vi "UHR-Fleezers Control (host) - 16.2.2v2.vi"() -> ()   [LabVIEW 2014] (continued)
            n3715 = Concatenate Strings("Lost tether (" ("Message to add"), w5032, " s)." ("string")) -> (w5034:string)
            n3716 = local write "Tether"(FALSE ("Tether")) -> ()
            n3717 = call "Update messages.vi"("Message to add"=w5034, "Old message string"=w5039) -> ("New message string"=w5038:string)
            n3718 = local write "Messages"(w5038) -> ()
            n3719 = property on="Fl. Triggered..." class="Bool (strict)"("Val(Sgnl)"=w5030) -> ()  [unwired: 2 in, 2 out]
            n3720 = local write "Dip for Protein"(w5030) -> ()
            n3721 = property on="Trap Pos. FB ON" class="Bool (strict)"("Val(Sgnl)"=w5030) -> ()  [unwired: 2 in, 2 out]
            n3722 = property on="Trap Trig. Fl." class="Bool (strict)"("Val(Sgnl)"=w5030) -> ()  [unwired: 2 in, 2 out]
          }
        }
      }
    }
    n3723 = case "For triggering actions based on the trap position (e.g., turning the excitation laser on if trap under feedback moves so far)" shown="True" "Trap Trig. Fl." {
      tunnel: w4490 -> [_ w4918]
      tunnel: w4503 -> [_ w4917]
      tunnel: ["" ("t") w4916] -> w4511
      tunnel: w4495 -> [_ w4915]
      tunnel: [0 ("t") w4914] -> w4508
      tunnel: w4507 -> [_ w4913]
      tunnel: w4482 -> [_ w4912]
      tunnel: w4481 -> [_ w4911]
      frame False {
      }
      frame True {
        n3724 = case shown="\"Wait for trigger\"" w4917 {
          tunnel: w4918 -> [w4935 _ _ w4983]
          tunnel: [w4932 w4964 "" ("t") w4986] -> w4916
          tunnel: w4915 -> [_ _ _ w4974]
          tunnel: [w4931 w4961 0 ("t") w4975] -> w4914
          tunnel: w4913 -> [_ w4963 _ w4981]
          tunnel: w4912 -> [w4920 w4958 _ w4977]
          tunnel: w4911 -> [w4919 w4957 _ w4976]
          frame "Wait for trigger" {
            n3725 = local read "Trap Trig. (FPGA)"() -> (w4923:bool)
            n3726 = Subtract(x=w4935, y="Mean T1 Position\nto compare (nm)") -> (x-y=w4928:dbl[])
            n3727 = call <vilib>:"Std Deviation and Variance.vi"("X"=w4928) -> ("mean"=→"mean":dbl, "standard deviation"=→"standard\ndeviation":dbl)  [unwired: 1 in, 1 out]
            n3728 = Array Max & Min(array=w4928) -> (max value=→"max value":dbl, min value=→"min value":dbl)  [unwired: 2 out]
            n3729 = Greater?(x=w4928, y="Threshold (nm)") -> (0:w4938:bool[])
            n3730 = case shown="True" w4923 {
              tunnel: w4920 -> [_ w4944]
              tunnel: w4919 -> [_ w4943]
              tunnel: [FALSE ("TTrig?") w4942] -> w4926
              frame False {
              }
              frame True {
                n3731 = xnode "Read/Write Control"("FPGA VI Reference In"=w4944, "error in"=w4943) -> ("TTrig?"=w4942:bool)  [unwired: 2 out]
              }
            }
            n3732 = Or Array Elements(Boolean array=w4938) -> (logical OR=w4925:bool)
            n3733 = Select(t=w4926, s=w4923, f=w4925) -> (s? t:f=w4924:bool)
            n3734 = Not(x=w4923) -> (.not. x?=w4922:bool)
            n3735 = And(x=w4924, y=w4922) -> (x .and. y?=w4921:bool)
            n3736 = Select(t="Triggered", s=w4924, f="Wait for trigger") -> (s? t:f=w4932:string)
            n3737 = case shown="True" w4924 {
              tunnel: [0 0] -> w4931
              tunnel: w4920 -> [_ w4949]
              tunnel: w4919 -> [_ w4948]
              frame False {
                "Waiting" <- TRUE ("Waiting")
              }
              frame True {
                n3738 = xnode "Read/Write Control"("FPGA VI Reference In"=w4949, "error in"=w4948, "TTrig?"=FALSE) -> ()  [unwired: 2 out]
                n3739 = local read "Messages"() -> (w4952:string)
                n3740 = call <vilib>:"Beep.vi"() -> ()  [unwired: 12 in]
                n3741 = call "Update messages.vi"("Message to add"="Unwinding trigger.", "Old message string"=w4952) -> ("New message string"=w4953:string)
                n3742 = local write "Messages"(w4953) -> ()
                n3743 = local write "Waiting"(FALSE ("Waiting")) -> ()
                "Triggered" <- TRUE ("Triggered")
              }
            }
            n3744 = case "Only need to turn on laser if host triggered" shown="True" w4921 {
              frame False {
              }
              frame True {
                n3745 = property on="Green Laser ON" class="Bool (strict)"("Val(Sgnl)"=TRUE ("Value (Signaling)")) -> ()  [unwired: 2 in, 2 out]
              }
            }
          }
          frame "Triggered" {
            n3746 = local read "Trap Trig. (FPGA)"() -> (w4960:bool)
            n3747 = Increment(x=w4963) -> (x+1=w4961:i32)
            n3748 = Greater Or Equal?(x=w4961, y="Fl. ON time (n)") -> (x >= y?=w4959:bool)
            n3749 = Select(t="Wait for trigger", s=w4959, f="Triggered" ("t")) -> (s? t:f=w4964:string)
            n3750 = And(x=w4959, y=w4960) -> (x .and. y?=w4956:bool)
            n3751 = case shown="True" w4956 {
              tunnel: w4958 -> [_ w4968]
              tunnel: w4957 -> [_ w4967]
              frame False {
              }
              frame True {
                n3752 = xnode "Read/Write Control"("FPGA VI Reference In"=w4968, "error in"=w4967, "FPGA Trap Trig"=TRUE) -> ()  [unwired: 2 out]
              }
            }
            n3753 = case shown="True" w4959 {
              frame False {
              }
              frame True {
                w4970 = FALSE ("Value (Signaling)")
                n3754 = local write "Triggered"(w4970) -> ()
                n3755 = local write "Waiting"(TRUE ("Waiting")) -> ()
                n3756 = property on="Green Laser ON" class="Bool (strict)"("Val(Sgnl)"=w4970) -> ()  [unwired: 2 in, 2 out]
              }
            }
          }
          frame "Do nothing" {
          }
          frame "Initialize", Default {
            n3757 = Increment(x=w4981) -> (x+1=w4985:i32)
            n3758 = Select(t=1, s=w4974, f=w4985) -> (s? t:f=w4975:i32)
            n3759 = feedback #29(w4983) -> (w4989:dbl[])
            n3760 = Build Array (concatenate)(w4983, w4989) -> (w4982:dbl[])
            n3761 = Greater Or Equal?(x=w4975, y="Wait to get offset (n)") -> (x >= y?=w4978:bool)
            n3762 = Select(t=w4983, s=w4974, f=w4982) -> (s? t:f=w4984:dbl[])
            n3763 = feedback-in #29(w4984) -> ()
            n3764 = call-poly <vilib>:"Mean.vi"("X"=w4984) -> ("mean"=w4979:dbl)  [unwired: 1 out]
            n3765 = local write "Mean T1 Position\nto compare (nm)"(w4979) -> ()
            n3766 = case shown="True" w4974 {
              tunnel: w4977 -> [_ w4995]
              tunnel: w4976 -> [_ w4994]
              frame False {
              }
              frame True {
                w4991 = FALSE ("FPGA Trap Trig")
                n3767 = xnode "Read/Write Control"("FPGA VI Reference In"=w4995, "error in"=w4994, "FPGA Trap Trig"=w4991) -> ("FPGA VI Reference Out"=w4993:T25, "error out"=w4992:errorcluster)
                n3768 = xnode "Read/Write Control"("FPGA VI Reference In"=w4993, "error in"=w4992, "TTrig?"=w4991) -> ()  [unwired: 2 out]
              }
            }
            n3769 = Select(t="Wait for trigger", s=w4978, f="Initialize") -> (s? t:f=w4986:string)
            n3770 = case shown="True" w4978 {
              tunnel: w4979 -> [_ w4998]
              tunnel: w4977 -> [_ w5007]
              tunnel: w4976 -> [_ w5006]
              frame False {
                n3771 = local write "Waiting"(FALSE ("Waiting")) -> ()
                "Initializing" <- TRUE ("Initializing")
              }
              frame True {
                n3772 = local read "Threshold (nm)"() -> (w5010:dbl)
                n3773 = local read "AOM X Cal (nm/MHz)"() -> (w5009:dbl)
                n3774 = Add(x=w4998, y=w5010) -> (x+y=w5011:dbl)
                n3775 = Divide(x=w5011, y=w5009) -> (x/y=w5008:dbl)
                n3776 = call "IR AOM freq to word.vi"("Frequency In (MHz)"=w5008) -> ("Frequency Word Out (double)"=w5005:dbl)
                n3777 = local write "Initializing"(FALSE ("Initializing")) -> ()
                n3778 = local write "Waiting"(TRUE ("Waiting")) -> ()
                n3779 = To Quad Integer(1:w5005) -> (0:w5004:i64)
                n3780 = xnode "Read/Write Control"("FPGA VI Reference In"=w5007, "error in"=w5006, "FPGA TTrig Thresh"=w5004) -> ("FPGA VI Reference Out"=w5001:T25, "error out"=w5000:errorcluster)
                n3781 = xnode "Read/Write Control"("FPGA VI Reference In"=w5001, "error in"=w5000, "FPGA Trap Trig"=TRUE) -> ()  [unwired: 2 out]
              }
            }
          }
        }
      }
    }
    n3782 = feedback-in #27(w4511) -> ()
    n3783 = feedback-in #28(w4508) -> ()
    n3784 = xnode ("Read/Write Control")("FPGA VI Reference In"=w4646, "error in"=w4645) -> ("FPGA VI Reference Out"=w4493:T25, "error out"=w4492:errorcluster, "AI2 Y Sum Set 1"=w4717:i16, "AI2 Y Sum Set 2"=w4716:i16, "AI1 X Set 1"=w4557:fxp<+/-,16,1>, "AI1 X Set 2"=w4556:fxp<+/-,16,1>, "Trap Pos FB Int Signal"=→"Trap Pos FB Int Signal":fxp<+/-,24,9>, "Trap Pos FB Int-Norm Signal"=→"Trap Pos FB Int-Norm Signal":fxp<+/-,16,1>, "Trap Pos FB Action"=w4550:i64, "Scanning"=→"AOD Scanning":bool, "Scan I"=→"AOD Scan I":u64, "Scanning MCL"=w4719:bool, "Scan I (MCL)"=→"MCL Scan I":u64, "Green FB Sum"=w4662:i16, "Trap Pos FB Action"=w4480:i64, "TTrig Fin Thresh"=w4476:i64, "Red FB Intensity"=w4460:i16, "Blue Intensity"=w4455:i16, "Random phase generated"=→"RF phase":fxp<+,14,14>)
    "MCL Scanning" <- w4719
    "Trap Pos FB Action" <- w4550
    n3785 = Divide(x=w4460, y=3276.7) -> (x/y=w4459:dbl)
    "Red laser intensity (V)" <- w4459
    n3786 = Divide(x=w4455, y=3276.7) -> (x/y=w4454:dbl)
    "Blue laser intensity (V)" <- w4454
    n3787 = Divide(x=w4662, y=3276.7) -> (x/y=w4458:dbl)
    "Green laser intensity (V)" <- w4458
    n3788 = local read "FB Trig Integrate"() -> (w4474:u32)
    n3789 = Divide(x=w4480, y=w4474) -> (x/y=w4473:dbl)
    "TTrig Sig (Int)" <- w4473
    n3790 = Bundle(w4458, w4459, w4454) -> (→"Fluorescence laser intensities plot":cluster{dbl, dbl, dbl})  [unwired: 1 in]
    n3791 = Divide(x=w4476, y=w4474) -> (x/y=w4471:dbl)
    "TTrig Fin Thresh (Int)" <- w4471
    n3792 = local read "AOM X Cal (nm/MHz)"() -> (w4479:dbl)
    n3793 = local read "AI2 (V)"() -> (w4718:cluster{"Set 1":dbl, "Set 2":dbl})
    n3794 = Bundle By Name(cluster=w4718, "Set 1"=w4717, "Set 2"=w4716) -> (w4714:cluster{"Set 1":dbl, "Set 2":dbl})
    n3795 = Divide(x=w4550, y=327.67) -> (x/y=→"Action (%)":dbl)
    n3796 = local read "Trap X (AI1)"() -> (w4570:T12)
    n3797 = call "IR AOM word double to freq.vi"("Frequency Word In (double)"=w4471) -> ("Frequency Out (MHz)"=w4470:dbl)
    n3798 = call "IR AOM word double to freq.vi"("Frequency Word In (double)"=w4473) -> ("Frequency Out (MHz)"=w4472:dbl)
    n3799 = Divide(x=w4714, y=3276.7) -> (x/y=w4713:cluster{"Set 1":dbl, "Set 2":dbl})
    n3800 = Multiply(x=w4472, y=w4479) -> (x*y=w4478:dbl)
    "TTrig Sig (nm)" <- w4478
    n3801 = Multiply(x=w4470, y=w4479) -> (x*y=w4477:dbl)
    "TTrig Fin Thresh (nm)" <- w4477
    n3802 = local write "AI2 (V)"(w4713) -> ()
    n3803 = Bundle(cluster=w4570, "Trap 1"=w4557, "Trap 2"=w4556) -> (→"Trap X (AI1)":T12)
    n3804 = Bundle(w4478, w4477) -> (→"TTrig":cluster{dbl, dbl})  [unwired: 1 in]
    n3805 = flat-sequence "To save data" {
      tunnel: [w5878] -> w4737
      tunnel: [w5879] -> w4736
      tunnel: w4690 -> [w5872]
      tunnel: w4498 -> [w5876]
      tunnel: ["Save Calibration"] -> w4710
      tunnel: w4707 -> [w5875]
      tunnel: [w5868] -> w4706
      tunnel: [w5865] -> w4705
      tunnel: [w5862] -> w4704
      tunnel: w4689 -> [w5864]
      tunnel: w4630 -> [w5858]
      tunnel: [w5858] -> w4629
      tunnel: [w5850] -> w4604
      tunnel: [w5853] -> w4538
      tunnel: [w5852] -> w4537
      tunnel: [w5846] -> w4392
      tunnel: w4737 -> [w6158]
      tunnel: w4736 -> [w6157]
      tunnel: w4539 -> [w6156]
      tunnel: w4710 -> [w6155]
      tunnel: w4706 -> [w6153]
      tunnel: w4705 -> [w6152]
      tunnel: w4704 -> [w6151]
      tunnel: w4611 -> [w6150]
      tunnel: w4638 -> [w6149]
      tunnel: w4629 -> [w6148]
      tunnel: w4604 -> [w6147]
      tunnel: w4399 -> [w6146]
      tunnel: w4441 -> [w6145]
      tunnel: w4538 -> [w6144]
      tunnel: w4537 -> [w6143]
      tunnel: w4536 -> [w6142]
      tunnel: w4462 -> [w6141]
      tunnel: w4390 -> [w6140]
      tunnel: w4392 -> [w6139]
      frame #0 {
        n3806 = Or(x="Start Saving", y="Start saving data + video") -> (x .or. y?=w5850:bool)
        n3807 = case shown="True" "Start saving data + video" {
          frame False {
          }
          frame True {
            n3808 = stacked-sequence {
              frame #0 {
                n3809 = local write "New Video File"(TRUE ("New Video File")) -> ()
              }
              frame #1 {
                n3810 = local write "Save Video"(TRUE ("Save Video")) -> ()
              }
            }
          }
        }
        n3811 = Or(x="Save N Sets", y=w5850) -> (x .or. y?=w5859:bool)
        n3812 = To Double Precision Float(number=w5875) -> (double precision float=w5869:dbl)
        n3813 = Build Array(w5859, "Save Calibration", w5872, w5864) -> (w5874:bool[])
        n3814 = Compound Arithmetic op=OR("Save Calibration", w5872, w5859, w5864) -> (w5877:bool)
        n3815 = Boolean Array To Number(Boolean array=w5874) -> (number=w5871:u32)
        n3816 = feedback #30(FALSE ("Save APD Data\nwith Trap Data")) -> (w5854:bool)
        n3817 = feedback #31(refnum<k0> refnum) -> (w5880:refnum<file>)
        n3818 = feedback #32(FALSE ("Save APD Data\nwith Trap Data")) -> (w5863:bool)
        n3819 = feedback #33(0) -> (w5882:i32)
        n3820 = feedback #34() -> (w5870:u32)  [unwired: 1 out]
        n3821 = feedback #35(refnum<k0> refnum) -> (w5847:refnum<file>)
        n3822 = feedback #36(refnum<k0> refnum) -> (w5856:refnum<file>)
        n3823 = feedback #37(refnum<k0> refnum) -> (w5866:refnum<file>)
        n3824 = case shown="True" w5877 {
          tunnel: [w5892 1] -> w5878
          tunnel: w5882 -> [w5894 _]
          tunnel: [w5893 w5927] -> w5879
          tunnel: w5880 -> [w5893 _]
          tunnel: w5876 -> [_ w5945]
          tunnel: w5869 -> [_ w5943]
          tunnel: w5871 -> [_ w5946]
          tunnel: [w5891 w5926] -> w5868
          tunnel: w5870 -> [w5891 _]
          tunnel: [w5890 w5924] -> w5865
          tunnel: w5866 -> [w5890 _]
          tunnel: [w5889 w5923] -> w5862
          tunnel: w5863 -> [w5889 _]
          tunnel: w5850 -> [_ w5921]
          tunnel: w5858 -> [_ w5920]
          tunnel: [w5888 w5912] -> w5852
          tunnel: w5856 -> [w5888 _]
          tunnel: [w5887 w5911] -> w5853
          tunnel: w5854 -> [w5887 _]
          tunnel: [w5886 w5895] -> w5846
          tunnel: w5847 -> [w5886 _]
          frame False {
            n3825 = Increment(x=w5894) -> (x+1=w5892:i32)
          }
          frame True {
            w5917 = FALSE ("Start Saving")
            w5922 = 9.0  # File Version
            w5929 = FALSE ("prepend array or string size? (T)")
            w5928 = T34."big-endian, network order" ("byte order (0:big-endian, network order)")
            # "Save trap position\ndata"
            n3826 = local read "BD 1 Frequency 1 (MHz)"() -> (w5942:dbl)
            n3827 = local read "BD 2 Frequency 1 (MHz)"() -> (w5941:dbl)
            n3828 = local read "BD 1 Frequency 2 (MHz)"() -> (w5940:dbl)
            n3829 = local read "BD 2 Frequency 2 (MHz)"() -> (w5939:dbl)
            n3830 = local read "BD 1 Frequency 3 (MHz)"() -> (w5938:dbl)
            n3831 = local read "BD 2 Frequency 3 (MHz)"() -> (w5937:dbl)
            n3832 = Array Size(array=w5920) -> (size(s)=w5919:i32)
            n3833 = To Double Precision Float(number=w5919) -> (double precision float=w5918:dbl)
            n3834 = local write "Save Calibration"(w5917) -> ()
            n3835 = local write "Start Saving"(w5917) -> ()
            n3836 = Build Array("Save APD Data\nwith Trap Data", "Save Trap Pos. Data") -> (w5914:bool[])
            n3837 = Boolean Array To Number(Boolean array=w5914) -> (number=w5913:u32)
            n3838 = Build Array(w5942, w5941, w5940, w5939, w5938, w5937) -> (w5936:dbl[])
            n3839 = case shown="2" w5946 {
              tunnel: w5945 -> [w6036 w6063 w6079 w6117]
              tunnel: w5918 -> [w6041 w6070 w6099 w6136]
              tunnel: w5943 -> [w6040 w6069 w6098 w6135]
              tunnel: [w6037 w6065 w6090 w6127] -> w5934
              tunnel: [w6028 "Cal sets to save" w6080 w6118] -> w5926
              tunnel: w5936 -> [w6038 w6066 w6092 w6129]
              tunnel: "Save APD Data\nwith Trap Data" -> [w6035 w6052 w6076 w6115]
              tunnel: [w6035 w6050 w6076 w6115] -> w5923
              tunnel: w5922 -> [w6031 w6059 w6074 w6113]
              tunnel: w5921 -> [w6030 _ _ _]
              tunnel: [w6021 w6058 w6073 w6103] -> w5911
              tunnel: "Save Trap Pos. Data" -> [w6021 w6057 w6073 w6103]
              tunnel: w5913 -> [w6020 w6056 w6072 w6102]
              frame 1, Default {
                # "timeseries"
                n3840 = case shown="False" "Profile" {
                  tunnel: [w6044 w6048] -> w6025
                  tunnel: [w6044 w6047] -> w6024
                  tunnel: [w6044 w6046] -> w6023
                  tunnel: [w6044 w6045] -> w6022
                  frame False {
                    w6044 = 0.0 ("f")
                  }
                  frame True {
                    n3841 = local read "Current Position"() -> (w6049:cluster{dbl, dbl, dbl})
                    n3842 = local read "Y change (mm)"() -> (w6045:dbl)
                    n3843 = Unbundle(w6049) -> (w6048:dbl, w6047:dbl, w6046:dbl)
                  }
                }
                n3844 = local read "Save ave N"() -> (w6043:dbl)
                n3845 = Multiply(x=w6043, y=w6036) -> (x*y=w6042:dbl)
                n3846 = To Double Precision Float(number=w6020) -> (double precision float=w6034:dbl)
                n3847 = Build Array(w6031, w6036, w6042, w6041, w6040, 0.0 ("f")) -> (w6039:dbl[])
                n3848 = Build Array(w6034, w6025, w6024, w6023, w6022) -> (w6032:dbl[])
                n3849 = Select(t=u32 4000000000, s=w6030, f="N sets to save") -> (s? t:f=w6028:u32)
                n3850 = Build Array (concatenate)(w6039, w6038, w6032) -> (w6037:dbl[])
              }
              frame 2 {
                w6061 = 0.0 ("f")
                w6051 = FALSE ("Save APD Data\nwith Trap Data")
                # "For diagnostics save trap position\ndata during cal"
                # "calibration"
                n3851 = Boolean To (0,1)(Boolean=w6051) -> (0, 1=w6055:i16)
                n3852 = Select(t=w6052, s="Save trap pos with cal", f=w6051) -> (s? t:f=w6050:bool)
                n3853 = Select(t=w6057, s="Save trap pos with cal", f=w6051) -> (s? t:f=w6058:bool)
                n3854 = Select(t=w6056, s="Save trap pos with cal", f=w6055) -> (s? t:f=w6054:u32)
                n3855 = To Double Precision Float(number=w6054) -> (double precision float=w6062:dbl)
                n3856 = Build Array(w6059, w6063, w6063, w6070, w6069, 1.0 ("t")) -> (w6067:dbl[])
                n3857 = Build Array(w6062, w6061, w6061, w6061, w6061) -> (w6060:dbl[])
                n3858 = Build Array (concatenate)(w6067, w6066, w6060) -> (w6065:dbl[])
                "Calibrating Trap..." <- TRUE ("Calibrating...")
              }
              frame 4 {
                w6077 = 0.0 ("f")
                # "scan dir (x/y = 0/1)"
                # "cycles/step"
                # "n scans (f/b)"
                # "steps"
                # "freq. range"
                # "AOD raster scan"
                n3859 = local read "Number of F/B Scans (AOD)"() -> (w6084:u16)
                n3860 = local read "Cycles/step (AOD)"() -> (w6086:u64)
                n3861 = local read "Scan Range (MHz)"() -> (w6089:dbl)
                n3862 = local read "Scan steps (AOD)"() -> (w6088:u64)
                n3863 = local read "Scan BD"() -> (w6096:bool)
                n3864 = local read "Save ave N"() -> (w6101:dbl)
                n3865 = Boolean To (0,1)(Boolean=w6096) -> (0, 1=w6095:i16)
                n3866 = To Double Precision Float(number=w6084) -> (double precision float=w6083:dbl)
                n3867 = To Double Precision Float(number=w6088) -> (double precision float=w6087:dbl)
                n3868 = To Double Precision Float(number=w6086) -> (double precision float=w6085:dbl)
                n3869 = To Double Precision Float(number=w6095) -> (double precision float=w6094:dbl)
                n3870 = Multiply(x=w6101, y=w6079) -> (x*y=w6100:dbl)
                n3871 = To Double Precision Float(number=w6072) -> (double precision float=w6078:dbl)
                n3872 = Build Array(w6078, w6077, w6077, w6077, w6077) -> (w6075:dbl[])
                n3873 = local read "N sets should be saved"() -> (w6081:dbl)
                n3874 = Build Array(w6094, w6089, w6087, w6085, w6083) -> (w6091:dbl[])
                n3875 = Build Array(w6074, w6079, w6100, w6099, w6098, 2.0 ("t")) -> (w6093:dbl[])
                n3876 = Round Toward +Infinity(x=w6081) -> (ceil(x): smallest int >= x=w6082:dbl)
                n3877 = Build Array (concatenate)(w6093, w6092, w6075, w6091) -> (w6090:dbl[])
                n3878 = To Unsigned Long Integer(number=w6082) -> (unsigned 32bit integer=w6080:u32)
              }
              frame 8 {
                w6110 = 0.0 ("f")
                # "MCL raster scan"
                n3879 = local read "Number of scans (MCL)"() -> (w6105:u64)
                n3880 = local read "Scan lines (y)"() -> (w6104:u64)
                n3881 = local read "2D or 1D Scan"() -> (w6107:bool)
                n3882 = local read "Scan Range (V)\n(of steps)"() -> (w6126:dbl)
                n3883 = local read "Fast Scan Dir"() -> (w6133:bool)
                n3884 = local read "Cycles/step (MCL)"() -> (w6123:u64)
                n3885 = local read "Scan steps (MCL)"() -> (w6125:u64)
                n3886 = Select(t=w6104, s=w6107, f=w6105) -> (s? t:f=w6106:u64)
                n3887 = Boolean To (0,1)(Boolean=w6107) -> (0, 1=w6109:i16)
                n3888 = local read "Save ave N"() -> (w6138:dbl)
                n3889 = local read "Initial X"() -> (w6112:dbl)
                n3890 = local read "Initial Y"() -> (w6111:dbl)
                n3891 = To Double Precision Float(number=w6109) -> (double precision float=w6108:dbl)
                n3892 = Boolean To (0,1)(Boolean=w6133) -> (0, 1=w6132:i16)
                n3893 = To Double Precision Float(number=w6106) -> (double precision float=w6121:dbl)
                n3894 = To Double Precision Float(number=w6125) -> (double precision float=w6124:dbl)
                n3895 = To Double Precision Float(number=w6123) -> (double precision float=w6122:dbl)
                n3896 = To Double Precision Float(number=w6132) -> (double precision float=w6131:dbl)
                n3897 = Multiply(x=w6138, y=w6117) -> (x*y=w6137:dbl)
                n3898 = To Double Precision Float(number=w6102) -> (double precision float=w6116:dbl)
                n3899 = local read "N sets should be saved (MCL)"() -> (w6119:dbl)
                n3900 = Build Array(w6116, w6108, w6110, w6110, w6110) -> (w6114:dbl[])
                n3901 = Build Array(w6131, w6126, w6124, w6122, w6121, w6112, w6111) -> (w6128:dbl[])
                n3902 = Build Array(w6113, w6117, w6137, w6136, w6135, 3.0 ("t")) -> (w6130:dbl[])
                n3903 = Round Toward +Infinity(x=w6119) -> (ceil(x): smallest int >= x=w6120:dbl)
                n3904 = Build Array (concatenate)(w6130, w6129, w6114, w6128) -> (w6127:dbl[])
                n3905 = To Unsigned Long Integer(number=w6120) -> (unsigned 32bit integer=w6118:u32)
              }
            }
            n3906 = local read "Index"() -> (w5951:dbl)
            n3907 = call "Create new save file.vi"("Insert"="", "Ext"=".dat", "Index In"=w5951) -> ("Path Out"=w5897:path, "Index Out"=w5925:dbl)
            n3908 = local write "Save file name"(w5897) -> ()
            n3909 = local write "Index"(w5925) -> ()
            n3910 = local write "Save index"(w5925) -> ()
            n3911 = case shown="True" "Save Event Log?" {
              tunnel: w5897 -> [_ w5959]
              tunnel: [refnum<k0> refnum w5958] -> w5895
              frame False {
              }
              frame True {
                (unwired) FALSE ("prepend array or string size? (T)")
                n3912 = Path To String(path=w5959) -> (string=w5970:string)
                n3913 = String Length(string=w5970) -> (length=w5969:i32)
                n3914 = Subtract(x=w5969, y=4) -> (x-y=w5967:i32)
                n3915 = String Subset(string=w5970, length (rest)=w5967) -> (substring=w5966:string)  [unwired: 1 out]
                n3916 = Concatenate Strings(w5966, "_log.txt" ("string")) -> (w5964:string)
                n3917 = String To Path(string=w5964) -> (path=w5960:path)
                n3918 = Open/Create/Replace File(file path (use dialog)=w5960, operation (0:open)=T35."create", access (0:read/write)=enum16{"read/write", "read-only", "write-only"}."write-only") -> (refnum out=w5961:refnum<file>)  [unwired: 1 in, 4 out]
                n3919 = Deny Access(7:w5961) -> (3:w5958:refnum<file>)  [unwired: 1 in, 2 out]
                n3920 = call "write to event log.vi"("log file ref"=w5958, "time"=0.0, "input string"="start log") -> ()  [unwired: 8 in]
              }
            }
            "log file ref" <- w5895
            n3921 = Array Size(array=w5934) -> (size(s)=w5935:i32)
            n3922 = Open/Create/Replace File(file path (use dialog)=w5897, operation (0:open)=T35."create", access (0:read/write)=enum16{"read/write", "read-only", "write-only"}."write-only") -> (refnum out=w5948:refnum<file>)  [unwired: 1 in, 4 out]
            n3923 = local write "Saving..."(TRUE ("Saving...")) -> ()
            n3924 = To Double Precision Float(number=w5935) -> (double precision float=w5933:dbl)
            n3925 = String Length(string="Comment (data description)") -> (length=w5932:i32)
            n3926 = To Double Precision Float(number=w5932) -> (double precision float=w5931:dbl)
            n3927 = Deny Access(7:w5948) -> (3:w5947:refnum<file>)  [unwired: 1 in, 2 out]
            n3928 = Build Array (concatenate)(w5933, w5934, w5931) -> (w5907:dbl[])
            n3929 = case "If fluorescence data to be saved" shown="True" w5923 {
              tunnel: w5897 -> [_ w6019]
              tunnel: [refnum<k0> refnum w5999] -> w5924
              frame False {
              }
              frame True {
                w5998 = 0.0
                n3930 = local read "APD host processing integration"() -> (w5994:dbl)
                n3931 = local read "APD Integration Time (s)"() -> (w6004:dbl)
                n3932 = local read "N APD Samp/step"() -> (w5997:dbl)
                n3933 = local read "Number of APDs"() -> (w5996:u8)
                n3934 = Path To String(path=w6019) -> (string=w6018:string)
                n3935 = String Length(string=w6018) -> (length=w6017:i32)
                n3936 = Subtract(x=w6017, y=4) -> (x-y=w6015:i32)
                n3937 = Multiply(x=w5997, y=w5994) -> (x*y=w5995:dbl)
                n3938 = String Subset(string=w6018, length (rest)=w6015) -> (substring=w6014:string)  [unwired: 1 out]
                n3939 = Build Array(w6004, w5995, w5996, w5998, w5998, w5998, w5998, w5998) -> (w6001:dbl[])
                n3940 = Concatenate Strings(w6014, "_fl.dat" ("string")) -> (w6012:string)
                n3941 = Array Size(array=w6001) -> (size(s)=w6003:i32)
                n3942 = String To Path(string=w6012) -> (path=w6008:path)
                n3943 = Open/Create/Replace File(file path (use dialog)=w6008, operation (0:open)=T35."create", access (0:read/write)=enum16{"read/write", "read-only", "write-only"}."write-only") -> (refnum out=w6009:refnum<file>)  [unwired: 1 in, 4 out]
                n3944 = Deny Access(7:w6009) -> (3:w6005:refnum<file>)  [unwired: 1 in, 2 out]
                n3945 = To Double Precision Float(number=w6003) -> (double precision float=w6002:dbl)
                n3946 = Build Array (concatenate)(w6002, w6001) -> (w6000:dbl[])
                n3947 = Write to Binary File(file (use dialog)=w6005, data=w6000, 5:FALSE ("prepend array or string size? (T)"), 9:T34."big-endian, network order" ("byte order (0:big-endian, network order)")) -> (refnum out=w5999:refnum<file>)  [unwired: 1 in, 3 out]
              }
            }
            n3948 = case shown="True" w5911 {
              tunnel: w5897 -> [_ w5978]
              tunnel: [refnum<k0> refnum w5977] -> w5912
              frame False {
              }
              frame True {
                w5973 = 0.0 ("element")
                n3949 = Path To String(path=w5978) -> (string=w5992:string)
                n3950 = Build Array(w5973, w5973, w5973, w5973, w5973, w5973, w5973, w5973) -> (w5974:dbl[])
                n3951 = String Length(string=w5992) -> (length=w5991:i32)
                n3952 = Subtract(x=w5991, y=4) -> (x-y=w5989:i32)
                n3953 = Array Size(array=w5974) -> (size(s)=w5976:i32)
                n3954 = String Subset(string=w5992, length (rest)=w5989) -> (substring=w5988:string)  [unwired: 1 out]
                n3955 = To Double Precision Float(number=w5976) -> (double precision float=w5975:dbl)
                n3956 = Concatenate Strings(w5988, "_pos.dat" ("string")) -> (w5986:string)
                n3957 = Build Array (concatenate)(w5975, w5974) -> (w5972:dbl[])
                n3958 = String To Path(string=w5986) -> (path=w5982:path)
                n3959 = Open/Create/Replace File(file path (use dialog)=w5982, operation (0:open)=T35."create", access (0:read/write)=enum16{"read/write", "read-only", "write-only"}."write-only") -> (refnum out=w5983:refnum<file>)  [unwired: 1 in, 4 out]
                n3960 = Deny Access(7:w5983) -> (3:w5979:refnum<file>)  [unwired: 1 in, 2 out]
                n3961 = Write to Binary File(file (use dialog)=w5979, data=w5972, 5:FALSE ("prepend array or string size? (T)"), 9:T34."big-endian, network order" ("byte order (0:big-endian, network order)")) -> (refnum out=w5977:refnum<file>)  [unwired: 1 in, 3 out]
              }
            }
            n3962 = Write to Binary File(file (use dialog)=w5947, data=w5907, 5:w5929, 9:w5928) -> (refnum out=w5930:refnum<file>)  [unwired: 1 in, 3 out]
            n3963 = Write to Binary File(file (use dialog)=w5930, data="Comment (data description)", 5:w5929, 9:w5928) -> (refnum out=w5927:refnum<file>)  [unwired: 1 in, 3 out]
            n3964 = local read "connection reference"() -> (w5909:T19)
            n3965 = Bundle("Comment (data description)"="Comment (data description)", "Channel 1 Buffer"="Channel 1 Buffer", "Channel 2 Buffer"="Channel 2 Buffer", "Channel 3 Buffer"="Channel 3 Buffer", "Title"="Title", "DNA Construct"="DNA Construct", "Bead diameter"="Bead diameter", "Name"="Name") -> (w5898:T59)  [unwired: 1 in]
            n3966 = call "MattFileCreator-v9.vi"("Comments"=w5898, "Input Array"=w5907, "File path"=w5897, "table"="labview", "connection reference"=w5909) -> ("connection reference out"=w5908:T19)  [unwired: 5 in, 1 out]
            n3967 = local write "connection reference"(w5908) -> ()
          }
        }
        n3968 = feedback-in #30(w5853) -> ()
        n3969 = feedback-in #31(w5879) -> ()
        n3970 = feedback-in #32(w5862) -> ()
        n3971 = feedback-in #33(w5878) -> ()
        n3972 = feedback-in #34(w5868) -> ()
        n3973 = feedback-in #35(w5846) -> ()
        n3974 = feedback-in #36(w5852) -> ()
        n3975 = feedback-in #37(w5865) -> ()
      }
      frame #1 {
        n3976 = local read "Saving..."() -> (w6154:bool)
        n3977 = case shown="True" w6154 {
          tunnel: w6158 -> [_ w6172]
          tunnel: w6157 -> [_ w6186]
          tunnel: w6156 -> [_ w6182]
          tunnel: w6155 -> [_ w6181]
          tunnel: w6153 -> [_ w6180]
          tunnel: w6152 -> [_ w6175]
          tunnel: w6151 -> [_ w6174]
          tunnel: w6150 -> [_ w6173]
          tunnel: w6149 -> [_ w6171]
          tunnel: w6148 -> [_ w6169]
          tunnel: w6147 -> [_ w6168]
          tunnel: w6146 -> [_ w6167]
          tunnel: w6145 -> [_ w6166]
          tunnel: w6144 -> [_ w6165]
          tunnel: w6143 -> [_ w6164]
          tunnel: w6142 -> [_ w6163]
          tunnel: w6141 -> [_ w6162]
          tunnel: w6140 -> [_ w6160]
          tunnel: w6139 -> [_ w6159]
          frame False {
          }
          frame True {
            n3978 = case shown="True" "Stop saving data + video" {
              frame False {
              }
              frame True {
                n3979 = local write "Save Video"(FALSE ("Save Video")) -> ()
              }
            }
            n3980 = Multiply(x=w6172, y=w6171) -> (x*y=→"Time (s)":dbl)
            n3981 = Less Or Equal?(x=w6172, y=w6180) -> (x <= y?=w6184:bool)
            n3982 = Compound Arithmetic op=OR("Stop Saving", "Abort save 2", "Stop saving data + video") -> (w6176:bool)
            n3983 = Not(x=w6176) -> (.not. x?=w6185:bool)
            n3984 = And(x=w6184, y=w6185) -> (x .and. y?=w6183:bool)
            n3985 = case shown="True" w6183 {
              tunnel: w6186 -> [w6196 w6295]
              tunnel: [0.0 w6298] -> w6179
              tunnel: w6172 -> [_ w6296]
              tunnel: w6180 -> [_ w6297]
              tunnel: w6182 -> [_ w6292]
              tunnel: w6181 -> [_ _]
              tunnel: w6175 -> [w6194 w6285]
              tunnel: w6174 -> [w6193 w6286]
              tunnel: w6173 -> [_ w6284]
              tunnel: w6169 -> [_ w6283]
              tunnel: w6168 -> [_ w6201]
              tunnel: w6167 -> [_ w6276]
              tunnel: w6166 -> [_ w6223]
              tunnel: w6165 -> [w6190 w6240]
              tunnel: w6164 -> [w6191 w6239]
              tunnel: w6163 -> [_ w6236]
              tunnel: w6162 -> [_ w6234]
              tunnel: w6160 -> [_ w6200]
              tunnel: w6159 -> [w6189 _]
              frame False {
                w6192 = FALSE
                n3986 = Close File(refnum=w6196) -> ()  [unwired: 1 in, 2 out]
                n3987 = case shown="True" w6193 {
                  tunnel: w6194 -> [_ w6199]
                  frame False {
                  }
                  frame True {
                    n3988 = Close File(refnum=w6199) -> ()  [unwired: 1 in, 2 out]
                  }
                }
                n3989 = case shown="True" w6190 {
                  tunnel: w6191 -> [_ w6198]
                  frame False {
                  }
                  frame True {
                    n3990 = Close File(refnum=w6198) -> ()  [unwired: 1 in, 2 out]
                  }
                }
                n3991 = local read "Save Event Log?"() -> (w6188:bool)
                n3992 = case shown="True" w6188 {
                  tunnel: w6189 -> [_ w6197]
                  frame False {
                  }
                  frame True {
                    n3993 = Close File(refnum=w6197) -> ()  [unwired: 1 in, 2 out]
                  }
                }
                n3994 = local write "Raster Scanning..."(w6192) -> ()
                n3995 = local write "Calibrating Trap..."(w6192) -> ()
                n3996 = call <vilib>:"Beep.vi"() -> ()  [unwired: 3 in, 9 out]
                n3997 = local write "Stop Saving"(w6192) -> ()
                "Saving..." <- w6192
              }
              frame True {
                n3998 = local read "Calibrating Trap..."() -> (w6287:bool)
                n3999 = case "Write fl. data" shown="True" w6286 {
                  tunnel: w6285 -> [_ w6321]
                  tunnel: w6284 -> [_ w6320]
                  frame False {
                  }
                  frame True {
                    n4000 = Write to Binary File(file (use dialog)=w6321, data=w6320, 5:FALSE ("prepend array or string size? (T)"), 9:T34."big-endian, network order" ("byte order (0:big-endian, network order)")) -> ()  [unwired: 1 in, 4 out]
                  }
                }
                n4001 = Greater?(x="Save ave N", y=1.0) -> (0:w6290:bool)
                n4002 = Not(x=w6287) -> (.not. x?=w6289:bool)
                n4003 = And(x=w6289, y=w6290) -> (x .and. y?=w6237:bool)
                n4004 = case shown="True" w6237 {
                  tunnel: w6236 -> [w6301 w6312]
                  tunnel: [w6301 w6304] -> w6235
                  tunnel: "Save ave N" -> [_ w6305]
                  frame False {
                  }
                  frame True {
                    w6302 = 2 ("dimension size")
                    n4005 = Array Size(array=w6312) -> (size(s)=w6306:i32)
                    n4006 = Divide(x=w6306, y=w6302) -> (x/y=w6310:dbl)
                    n4007 = Reshape Array(w6312, w6310, w6302) -> (w6311:u64[][])
                    n4008 = Transpose 2D Array(2D array=w6311) -> (transposed array=w6309:u64[][])
                    n4009 = for {
                      tunnel: w6309 -> [w6314] mode=indexing
                      tunnel: [w6313] -> w6303 mode=indexing
                      tunnel: w6305 -> [w6315]
                      workers-P: _ -> [_]
                      n4010 = call "downsample 1D array - U64.vi"("Ave N"=w6315, "Array In"=w6314) -> ("Array Out"=w6313:u64[])  [unwired: 1 in]
                    }
                    n4011 = Transpose 2D Array(2D array=w6303) -> (transposed array=w6308:u64[][])
                    n4012 = Divide(x=w6306, y=w6305) -> (x/y=w6307:dbl)
                    n4013 = Reshape Array(w6308, w6307) -> (w6304:u64[])
                  }
                }
                n4014 = case shown="True" w6237 {
                  tunnel: w6292 -> [w6324 w6336]
                  tunnel: [w6324 w6328] -> w6288
                  tunnel: "Save ave N" -> [_ w6329]
                  tunnel: w6283 -> [_ w6327]
                  frame False {
                  }
                  frame True {
                    n4015 = Array Size(array=w6336) -> (size(s)=w6330:i32)
                    n4016 = Array Size(array=w6327) -> (size(s)=w6326:i32)
                    n4017 = Divide(x=w6330, y=w6326) -> (x/y=w6334:dbl)
                    n4018 = Reshape Array(w6336, w6334, w6326) -> (w6335:i16[][])
                    n4019 = Transpose 2D Array(2D array=w6335) -> (transposed array=w6333:i16[][])
                    n4020 = for {
                      tunnel: w6333 -> [w6339] mode=indexing
                      tunnel: [w6338] -> w6325 mode=indexing
                      tunnel: w6329 -> [w6337]
                      workers-P: _ -> [_]
                      n4021 = call "downsample 1D array - I16.vi"("Ave N"=w6337, "Array In"=w6339) -> ("Array Out"=w6338:i16[])  [unwired: 1 out]
                    }
                    n4022 = Transpose 2D Array(2D array=w6325) -> (transposed array=w6332:i16[][])
                    n4023 = Divide(x=w6330, y=w6329) -> (x/y=w6331:dbl)
                    n4024 = Reshape Array(w6332, w6331) -> (w6328:i16[])
                  }
                }
                n4025 = Index Array(array=w6223, index=2) -> (element=w6224:waveform(dbl))
                n4026 = Index Array(array=w6223, index=1) -> (element=w6257:waveform(dbl))
                n4027 = Index Array(array=w6223, index=0) -> (element=w6259:waveform(dbl))
                n4028 = Unbundle By Name(w6224) -> ("Y"=w6226:dbl[])
                n4029 = Unbundle By Name(w6257) -> ("Y"=w6261:dbl[])
                n4030 = Unbundle By Name(w6259) -> ("Y"=w6269:dbl[])
                n4031 = case "Write trap pos. data" shown="True" w6240 {
                  tunnel: w6239 -> [_ w6317]
                  tunnel: w6235 -> [_ w6316]
                  frame False {
                  }
                  frame True {
                    n4032 = Write to Binary File(file (use dialog)=w6317, data=w6316, 5:FALSE ("prepend array or string size? (T)"), 9:T34."big-endian, network order" ("byte order (0:big-endian, network order)")) -> ()  [unwired: 1 in, 4 out]
                  }
                }
                n4033 = Write to Binary File(file (use dialog)=w6295, data=w6288, 5:FALSE ("prepend array or string size? (T)"), 9:T34."big-endian, network order" ("byte order (0:big-endian, network order)")) -> ()  [unwired: 1 in, 4 out]
                n4034 = feedback #38(w6226) -> (w6227:dbl[])
                n4035 = Build Array (concatenate)(w6227, w6226) -> (w6222:dbl[])
                n4036 = Select(t=w6226, s=w6201, f=w6222) -> (s? t:f=w6212:dbl[])
                n4037 = feedback-in #38(w6212) -> ()
                n4038 = feedback #39(w6261) -> (w6263:dbl[])
                n4039 = Build Array (concatenate)(w6263, w6261) -> (w6262:dbl[])
                n4040 = Select(t=w6261, s=w6201, f=w6262) -> (s? t:f=w6251:dbl[])
                n4041 = feedback-in #39(w6251) -> ()
                n4042 = feedback #40(w6269) -> (w6282:dbl[])
                n4043 = Build Array (concatenate)(w6282, w6269) -> (w6281:dbl[])
                n4044 = Select(t=w6269, s=w6201, f=w6281) -> (s? t:f=w6256:dbl[])
                n4045 = feedback-in #40(w6256) -> ()
                n4046 = Divide(x=w6296, y=w6297) -> (x/y=w6299:dbl)
                n4047 = Multiply(x=w6299, y=100.0) -> (x*y=w6298:dbl)
                n4048 = Build Array(w6256, w6251, w6212) -> (→"Saved APD":dbl[][])
                n4049 = Array Size(array=w6256) -> (size(s)=w6274:i32)
                n4050 = Unbundle By Name(w6276) -> ("Y"=w6280:dbl[])
                n4051 = Subtract(x=w6274, y="N pts to average") -> (x-y=w6209:i32)
                n4052 = Multiply(x="N pts to average", y=u16 2) -> (x*y=w6252:u16)
                n4053 = Subtract(x=w6274, y=w6252) -> (x-y=w6210:i32)
                n4054 = feedback #41(w6280) -> (w6279:dbl[])
                n4055 = Build Array (concatenate)(w6279, w6280) -> (w6278:dbl[])
                n4056 = Select(t=w6280, s=w6201, f=w6278) -> (s? t:f=w6277:dbl[])
                "Trap Delta Graph" <- w6277
                n4057 = feedback-in #41(w6277) -> ()
                n4058 = Array Subset(array=w6256, index=w6209, length="N pts to average") -> (w6273:dbl[])
                n4059 = Array Subset(array=w6256, index=w6210, length="N pts to average") -> (w6272:dbl[])
                n4060 = Array Subset(array=w6251, index=w6209, length="N pts to average") -> (w6254:dbl[])
                n4061 = Array Subset(array=w6251, index=w6210, length="N pts to average") -> (w6253:dbl[])
                n4062 = Array Subset(array=w6212, index=w6209, length="N pts to average") -> (w6221:dbl[])
                n4063 = Array Subset(array=w6212, index=w6210, length="N pts to average") -> (w6220:dbl[])
                n4064 = Index Array(array=w6234, index=0) -> (element=w6232:waveform(dbl))
                n4065 = call-poly <vilib>:"Mean.vi"("X"=w6273) -> ("mean"=w6271:dbl)  [unwired: 1 out]
                n4066 = call-poly <vilib>:"Mean.vi"("X"=w6254) -> ("mean"=w6250:dbl)  [unwired: 1 out]
                n4067 = call-poly <vilib>:"Mean.vi"("X"=w6272) -> ("mean"=w6270:dbl)  [unwired: 1 out]
                n4068 = call-poly <vilib>:"Mean.vi"("X"=w6253) -> ("mean"=w6249:dbl)  [unwired: 1 out]
                n4069 = call-poly <vilib>:"Mean.vi"("X"=w6221) -> ("mean"=w6219:dbl)  [unwired: 1 out]
                n4070 = call-poly <vilib>:"Mean.vi"("X"=w6220) -> ("mean"=w6218:dbl)  [unwired: 1 out]
                n4071 = Unbundle By Name(w6232) -> ("Y"=w6230:dbl[])
                n4072 = Subtract(x=w6250, y=w6249) -> (x-y=w6241:dbl)
                "Delta Fl. 2" <- w6241
                n4073 = Subtract(x=w6219, y=w6218) -> (x-y=w6213:dbl)
                "Delta Fl. 3" <- w6213
                n4074 = Subtract(x=w6271, y=w6270) -> (x-y=w6268:dbl)
                "Delta Fl. 1" <- w6268
                n4075 = feedback #42(w6230) -> (w6229:dbl[])
                n4076 = Build Array (concatenate)(w6229, w6230) -> (w6231:dbl[])
                n4077 = Initialize Array(w6268, 1 ("dimension size")) -> (w6265:dbl[])
                n4078 = Initialize Array(w6241, 1 ("dimension size")) -> (w6246:dbl[])
                n4079 = Initialize Array(w6213, 1 ("dimension size")) -> (w6215:dbl[])
                n4080 = Select(t=w6230, s=w6201, f=w6231) -> (s? t:f=w6228:dbl[])
                "Saved trap pos" <- w6228
                n4081 = feedback-in #42(w6228) -> ()
                n4082 = feedback #43(w6265) -> (w6266:dbl[])
                n4083 = Build Array (concatenate)(w6266, w6265) -> (w6264:dbl[])
                n4084 = feedback #44(w6246) -> (w6247:dbl[])
                n4085 = feedback #45(w6215) -> (w6216:dbl[])
                n4086 = Build Array (concatenate)(w6247, w6246) -> (w6245:dbl[])
                n4087 = Build Array (concatenate)(w6216, w6215) -> (w6214:dbl[])
                n4088 = Select(t=w6265, s=w6201, f=w6264) -> (s? t:f=w6244:dbl[])
                n4089 = feedback-in #43(w6244) -> ()
                n4090 = Select(t=w6246, s=w6201, f=w6245) -> (s? t:f=w6243:dbl[])
                n4091 = feedback-in #44(w6243) -> ()
                n4092 = Select(t=w6215, s=w6201, f=w6214) -> (s? t:f=w6208:dbl[])
                n4093 = feedback-in #45(w6208) -> ()
                n4094 = Build Array(w6244, w6243, w6208) -> (→"Save APD Deriv":dbl[][])
                n4095 = Index Array(array=w6200, index=15) -> (element=w6206:waveform(dbl))
                n4096 = Unbundle By Name(w6206) -> ("Y"=w6204:dbl[])
                n4097 = feedback #46(w6204) -> (w6203:dbl[])
                n4098 = Build Array (concatenate)(w6203, w6204) -> (w6205:dbl[])
                n4099 = Select(t=w6204, s=w6201, f=w6205) -> (s? t:f=w6202:dbl[])
                "Amp current" <- w6202
                n4100 = feedback-in #46(w6202) -> ()
              }
            }
            "Progress" <- w6179
            "Progress 2" <- w6179
          }
        }
      }
    }
    n4101 = local read "wait to reset values"() -> (w4721:bool)
    n4102 = Not(x=w4719) -> (.not. x?=w4722:bool)
    n4103 = And(x=w4722, y=w4721) -> (x .and. y?=w4723:bool)
    n4104 = case "Part of MCL raster scanning: returns to initial positions after scan done" shown="True" w4723 {
      tunnel: w4493 -> [w5666 w5673]
      tunnel: [w5666 w5672] -> w4725
      tunnel: w4492 -> [w5665 w5671]
      tunnel: [w5665 w5670] -> w4720
      frame False {
      }
      frame True {
        w5681 = 10.0 ("y")
        w5680 = 32767.0 ("y")
        # "to return scan values\nafter a synchronous \nAOM scan"
        n4105 = local read "AO2"() -> (w5674:dbl)
        n4106 = local read "AO1"() -> (w5675:dbl)
        n4107 = local write "wait to reset values"(FALSE ("wait to reset values")) -> ()
        n4108 = Multiply(x=w5675, y=w5680) -> (x*y=w5677:dbl)
        n4109 = Multiply(x=w5674, y=w5680) -> (x*y=w5679:dbl)
        n4110 = Divide(x=w5677, y=w5681) -> (x/y=w5676:dbl)
        n4111 = Divide(x=w5679, y=w5681) -> (x/y=w5678:dbl)
        n4112 = To Word Integer(number=w5676) -> (16bit integer=w5682:i16)
        n4113 = To Word Integer(number=w5678) -> (16bit integer=w5683:i16)
        n4114 = local read "Total Counts (ticks)"() -> (w5667:u16)
        n4115 = xnode "Read/Write Control"("FPGA VI Reference In"=w5673, "error in"=w5671, "AO1"=w5682, "AO2"=w5683, "MCL count"=w5667) -> ("FPGA VI Reference Out"=w5672:T25, "error out"=w5670:errorcluster)
        n4116 = local read "Scan Range (V)\n(of steps)"() -> (w5668:dbl)
        n4117 = property on="Scan Range (V)\n(of steps)" class="DigNum (strict)"("Val(Sgnl)"=w5668) -> ()  [unwired: 2 in, 2 out]
      }
    }
    n4118 = case shown="True" "Sound ON" {
      tunnel: [w4794 w4839] -> w4423
      tunnel: w4422 -> [w4794 w4838]
      tunnel: w4420 -> [_ _]
      tunnel: w4398 -> [_ w4797]
      tunnel: w4419 -> [_ _]
      tunnel: w4418 -> [_ w4808]
      tunnel: w4417 -> [_ w4818]
      frame False {
      }
      frame True {
        n4119 = Index Array(array=w4797, index="Data channel to sound") -> (element=w4796:waveform(dbl))
        "Waveform Graph 2" <- w4796
        n4120 = Unbundle By Name(w4796) -> ("dt"=w4822:dbl, "Y"=w4820:dbl[])
        n4121 = Array Size(array=w4820) -> (size(s)=w4821:i32)
        "N data samples" <- w4821
        n4122 = for "Data time base" {
          N: w4821 -> [_]
          tunnel: [w4843] -> w4823 mode=indexing
          i -> [w4843]
        }
        n4123 = Multiply(x=w4822, y=w4823) -> (x*y=w4819:dbl[])
        n4124 = Compound Arithmetic op=MULTIPLY(6.283185307179586, "Carrier Frequency (Hz)", w4818) -> (w4835:dbl[])
        n4125 = call <vilib>:"Interpolate 1D.vi"("X is monotonic"=TRUE, "xi"=w4818, "X"=w4819, "Y"=w4820) -> ("yi"=w4816:dbl[])  [unwired: 5 in, 2 out]
        n4126 = Sine(x=w4835) -> (sin(x)=w4824:dbl[])
        n4127 = Add(x=w4816, y="Offset") -> (x+y=w4814:dbl[])
        n4128 = Multiply(x=w4814, y="mult x") -> (x*y=w4812:dbl[])
        n4129 = Add(x="Offset 2", y=w4812) -> (x+y=w4807:dbl[])
        n4130 = Compound Arithmetic op=MULTIPLY(6.283185307179586, "Carrier Frequency (Hz)", w4808, w4807) -> (w4799:dbl[])
        n4131 = for "Cumulative sum" {
          tunnel: [w4842] -> w4805 mode=indexing
          shift-right: [w4842] -> w4802
          shift-left: 0.0 -> [w4841]
          tunnel: w4799 -> [w4840] mode=indexing
          n4132 = Add(x=w4840, y=w4841) -> (x+y=w4842:dbl)
        }
        n4133 = feedback #47(0.0) -> (w4801:dbl)
        n4134 = Add(x=w4805, y=w4801) -> (x+y=w4804:dbl[])
        n4135 = Add(x=w4802, y=w4801) -> (x+y=w4800:dbl)
        n4136 = feedback-in #47(w4800) -> ()
        n4137 = Sine(x=w4804) -> (sin(x)=w4798:dbl[])
        n4138 = Select(t=w4824, s="tone or data", f=w4798) -> (s? t:f=w4830:dbl[])
        n4139 = Multiply(x=w4830, y="Volume") -> (x*y=w4828:dbl[])
        n4140 = Initialize Array(0.0 ("element"), "N initial buffer elements") -> (w4831:dbl[])
        n4141 = Multiply(x="N initial buffer elements", y=w4808) -> (x*y=→"Initial buffer time (s)":dbl)
        n4142 = Build Array (concatenate)(w4831, w4828) -> (w4833:dbl[])
        n4143 = First Call?() -> (First Call?: T/F=w4834:bool)
        n4144 = Select(t=w4833, s=w4834, f=w4828) -> (s? t:f=w4827:dbl[])
        n4145 = call-poly <vilib>:"Sound Output Write.vi"("data"=w4827, "task ID"=w4838) -> ("task ID out"=w4839:T44)  [unwired: 8 in, 1 out]
      }
    }
    n4146 = node-c288() -> ()  [unwired: 2 out]
  }
  n4147 = node-c288(w90) -> ()  [unwired: 1 out]
  n4148 = call <vilib>:"Sound Output Clear.vi"("task ID"=w31) -> ()  [unwired: 10 in, 1 out]
  n4149 = flat-sequence {
    tunnel: w97 -> [w6343]
    tunnel: w98 -> [w6344]
    tunnel: [w6342] -> w96
    tunnel: [w6341] -> w95
    tunnel: w94 -> [_]
    tunnel: w92 -> [_]
    tunnel: w88 -> [_]
    tunnel: w96 -> [w6345]
    tunnel: w95 -> [w6346]
    frame #0 {
      w6340 = FALSE ("AI to FIFO")
      n4150 = xnode "Read/Write Control"("FPGA VI Reference In"=w6344, "error in"=w6343, "AI to FIFO"=w6340, "APD to FIFO"=w6340) -> ("FPGA VI Reference Out"=w6342:T25, "error out"=w6341:errorcluster)
    }
    frame #1 {
      n4151 = xnode "Close FPGA VI Reference"("FPGA VI Reference In"=w6345, "error in"=w6346) -> ("error out"=→"error out":errorcluster)
    }
  }
